vi "CurrentVsTime.vi"() -> ()   [LabVIEW 2016]
uses:
  <vilib>/Analysis/baseanly.llb/Mean (DBL).vi
  <vilib>/Analysis/NI_AALBase.lvlib
panel:
  out "Elapsed Time (s)":dbl
  in  "Number of Samples":i32=1000
  in  "Measurement Time(s)":dbl=1.0 caption="Time Target (s)"
  in  "Voltage (V)":dbl
  in  "Filename":path=path "C:/Users/tysoe-lab/Desktop/1.lvm"
  in  "Comment":string
  out "Current vs. Time":cluster{"X":dbl[], "Y":dbl[]}[](graph)
  # "MEASUREMENT \nPARAMETERS"
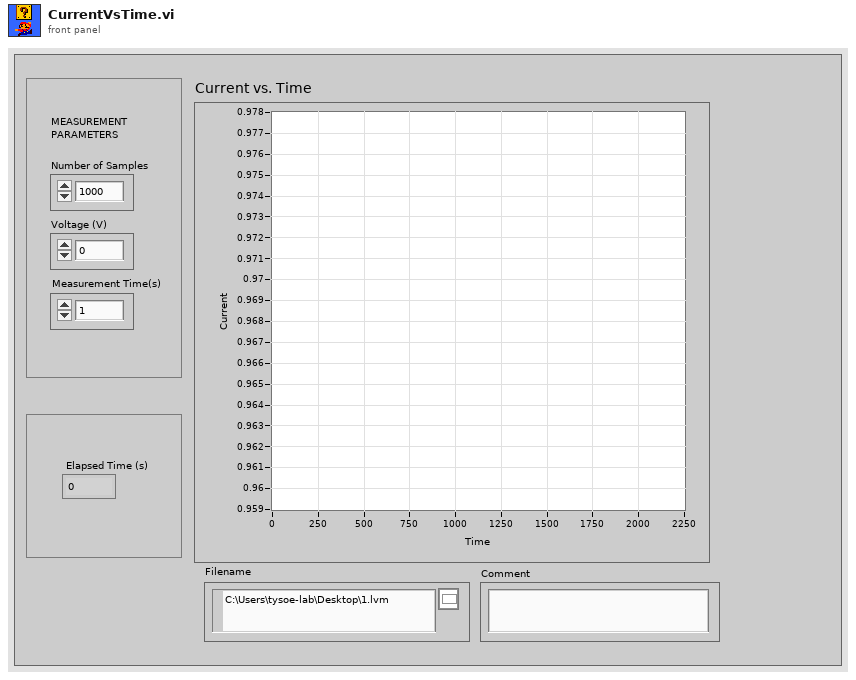
[diagram p1: front panel]
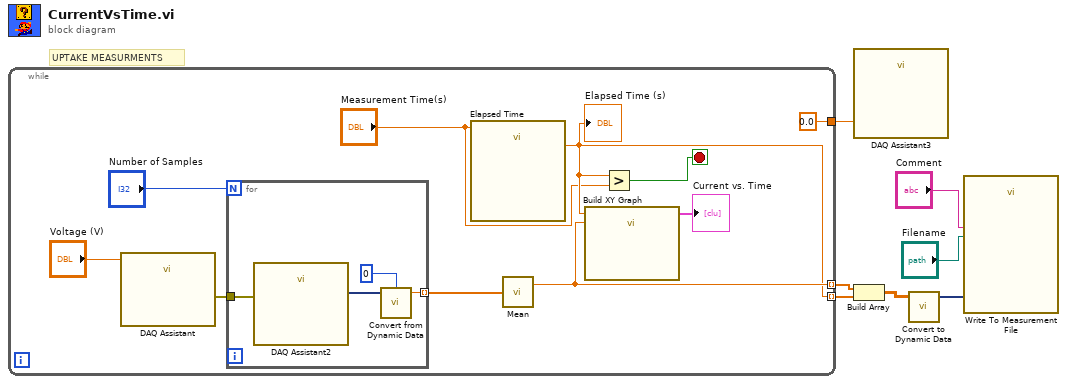
[diagram p0: block diagram]
diagram:
  # "UPTAKE MEASURMENTS"
  n1 = while {
    tunnel: [0.0 ("data")] -> w5
    tunnel: [w11] -> w4 mode=indexing
    tunnel: [w9] -> w3 mode=indexing
    stop <- w10 stop-if-true
    n2 = call "DAQ Assistant"("data"="Voltage (V)") -> ("error out"=w16:errorcluster)  [unwired: 17 in, 1 out]
    n3 = for {
      N: "Number of Samples" -> [_]
      tunnel: w16 -> [w21]
      tunnel: [w18] -> w12 mode=indexing
      n4 = call "DAQ Assistant2"("error in"=w21) -> ("data"=w19:dynamicdata)  [unwired: 16 in, 2 out]
      n5 = call "Convert from Dynamic Data"("Dynamic Data Type"=w19, "Channel"=0) -> ("Scalar"=w18:dbl)  [unwired: 2 in]
    }
    n6 = call "Elapsed Time"("Time Target (s)"="Measurement Time(s)") -> ("Elapsed Time (s)"=w9:dbl)  [unwired: 11 in, 7 out]
    "Elapsed Time (s)" <- w9
    n7 = call-poly <vilib>:"Mean.vi"("X"=w12) -> ("mean"=w11:dbl)  [unwired: 1 out]
    n8 = call "Build XY Graph"("Y Input"=w11, "X Input"=w9) -> ("XY Graph"=→"Current vs. Time":cluster{"X":dbl[], "Y":dbl[]}[])  [unwired: 8 in, 1 out]
    n9 = Greater?(x=w9, y="Measurement Time(s)") -> (0:w10:bool)
  }
  n10 = call "DAQ Assistant3"("data"=w5) -> ()  [unwired: 17 in, 2 out]
  n11 = Build Array(w4, w3) -> (w2:dbl[][])
  n12 = call "Convert to Dynamic Data"("2D Array"=w2) -> ("Dynamic Data Type"=w1:dynamicdata)  [unwired: 3 in]
  n13 = call "Write To Measurement File"("Signals"=w1, "Filename"="Filename", "Comment"="Comment") -> ()  [unwired: 14 in, 3 out]
